vi "Stacking SSI.vi"(10 "Stacking SS State":T3, 11 "Robot Controls":T4) -> (3 "Stacking Actuators Out":T1)   [LabVIEW 2014]
uses:
  Robot Commands.ctl
  Stacking SS State.ctl
  Stacking SS Actuators.ctl
  <vilib>/Rock Robotics/WPI/Solenoid/WPI_SolenoidValue.ctl
  Global Variables/Settings.vi
  Global Variables/Lifter Sequences.vi
panel:
  out "Totes in Bot":i32
  # "Field Centric"
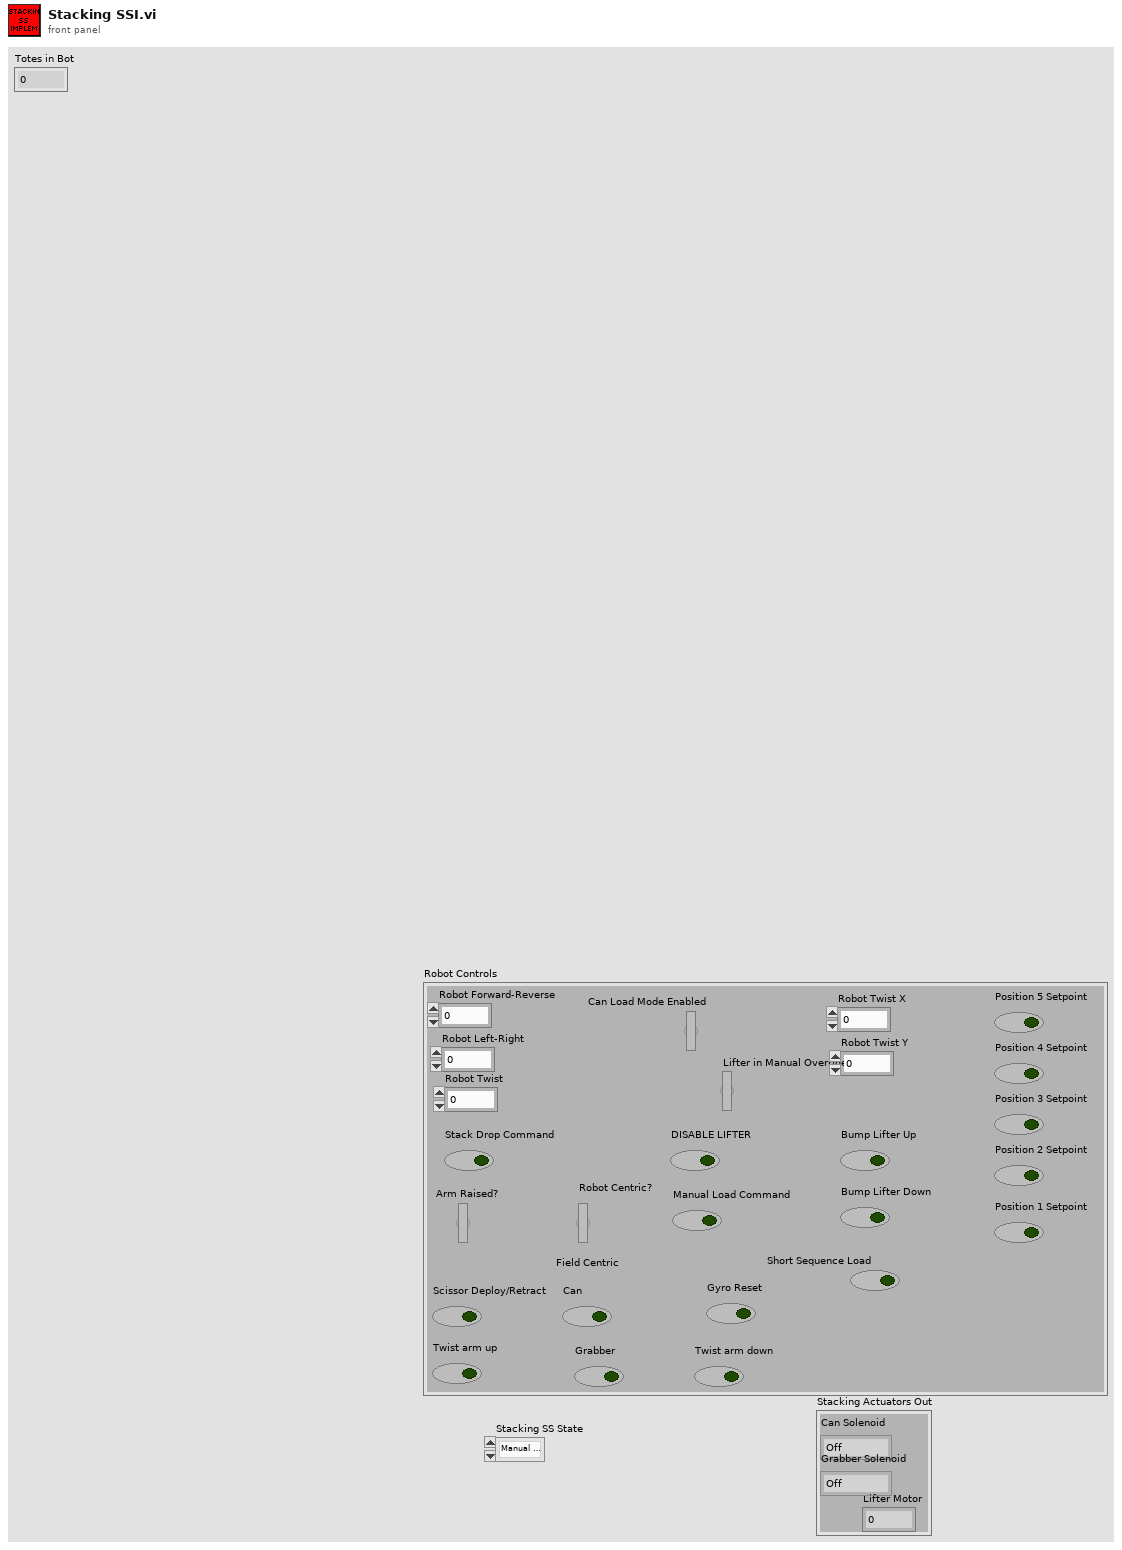
[diagram p1: front panel]
types:
  T1 = typedef "Stacking SS Actuators.ctl" = cluster{"Can Solenoid":T2, "Lifter Motor":dbl, "Grabber Solenoid":T2}
  T2 = typedef "WPI_SolenoidValue.ctl" = enum16{"Off", "On", "Forward", "Reverse"}
  T3 = typedef "Stacking SS State.ctl" = enum16{"Manual Load", "Manual Override"}
  T4 = typedef "Robot Commands.ctl" = cluster{"Robot Forward-Reverse":dbl, "Robot Left-Right":dbl, "Robot Twist":dbl, "Can Load Mode Enabled":bool, "Lifter in Manual Override?":bool, "Stack Drop Command":bool, "Arm Raised?":bool, "DISABLE LIFTER":bool, "Position 1 Setpoint":bool, "Position 2 Setpoint":bool, "Position 3 Setpoint":bool, "Position 4 Setpoint":bool, "Position 5 Setpoint":bool, "Bump Lifter Down":bool, "Bump Lifter Up":bool, "Manual Load Command":bool, "Robot Centric?":bool, "Scissor Deploy/Retract":bool, "Grabber":bool, "Can":bool, "Twist arm up":bool, "Gyro Reset":bool, "Twist arm down":bool, "Short Sequence Load":bool, "Robot Twist X":dbl, "Robot Twist Y":dbl}
  T5 = cluster{"Setpoint Commands":enum16{"No Op", "Setpoint 1", "Setpoint 2", "Setpoint 3", "Setpoint 4", "Setpoint 5"}[], "Setpoint Commands Wait for Input?":bool[], "Setpoint Commands Time Wait after setpoint reachd":i32[], "Can Solenoid Commands":enum16{"Disengaged", "Engaged"}[], "Grabber Solenoid Commands":enum16{"Disengaged", "Engaged"}[]}
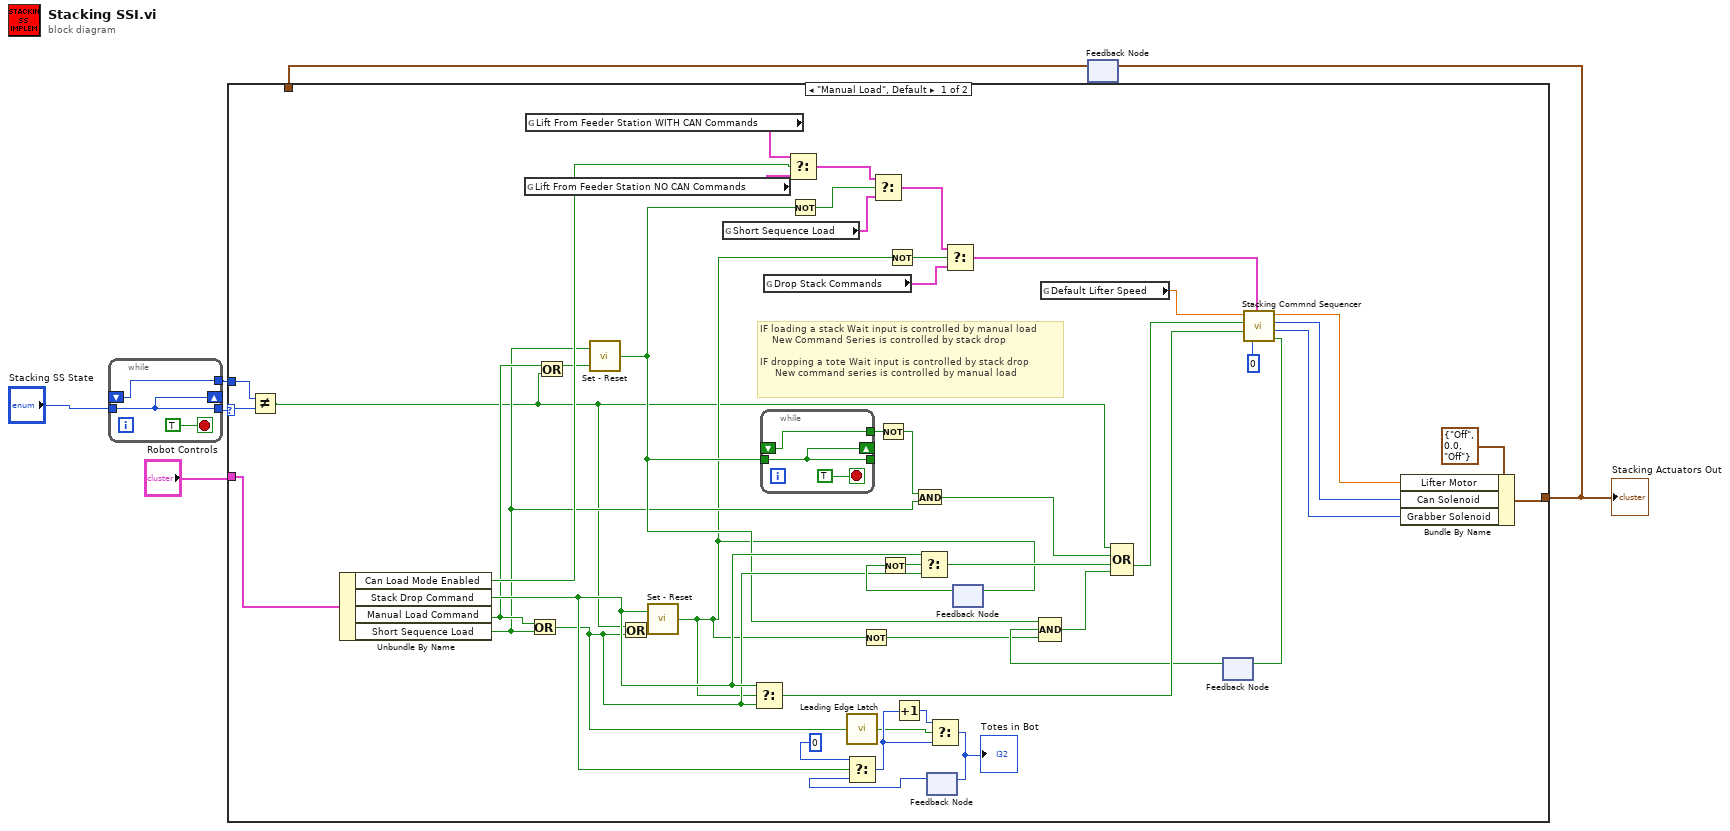
[diagram p0: block diagram]
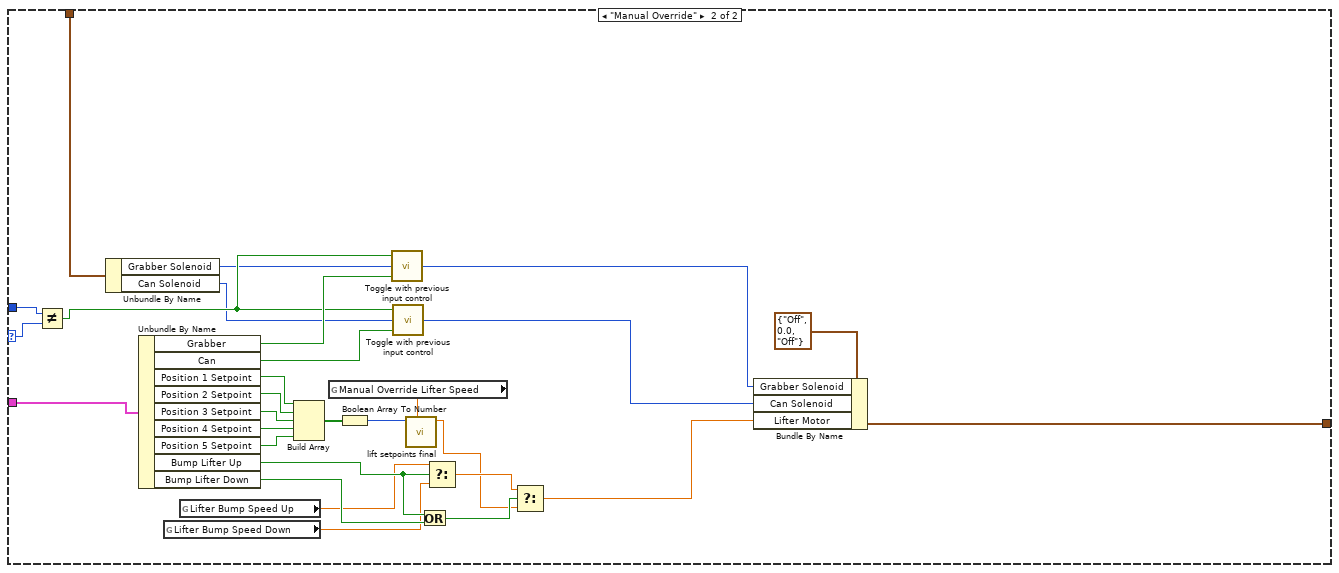
[diagram p2: hidden frame]
diagram:
  n1 = while {
    tunnel: "Stacking SS State" -> [w8]
    tunnel: [w8] -> w3
    shift-right: [w8] -> _
    shift-left: _ -> [w7]
    tunnel: [w7] -> w4
    stop <- TRUE stop-if-true
  }
  n2 = feedback #1() -> (w1:T1)  [unwired: 1 in]
  n3 = case shown="\"Manual Load\", Default" w3 {
    selector: w3 -> [w15 w67]
    tunnel: "Robot Controls" -> [w22 w88]
    tunnel: [w56 w74] -> w2
    tunnel: w4 -> [w14 w66]
    tunnel: w1 -> [_ w62]
    frame "Manual Load", Default {
      # "IF loading a stack Wait input is controlled by manual load\n    New Command Series is controlled by stack drop\n\nIF dropping a tote Wait input is controlled by stack drop\n     New command series is controlled by manual load"
      n4 = Not Equal?(x=w14, y=w15) -> (x != y?=w10:bool)
      n5 = Unbundle By Name(w22) -> ("Can Load Mode Enabled"=w53:bool, "Stack Drop Command"=w51:bool, "Manual Load Command"=w28:bool, "Short Sequence Load"=w25:bool)
      n6 = global read "Lifter Sequences.vi" "Lift From Feeder Station NO CAN Commands"() -> (w44:T5)
      n7 = global read "Lifter Sequences.vi" "Lift From Feeder Station WITH CAN Commands"() -> (w43:T5)
      n8 = Or(x=w28, y=w25) -> (x .or. y?=w36:bool)
      n9 = Or(x=w28, y=w10) -> (x .or. y?=w12:bool)
      n10 = call "Set - Reset.vi"("Reset"=w12, "Set"=w25) -> ("Output"=w26:bool)
      n11 = Or(x=w10, y=w36) -> (x .or. y?=w11:bool)
      n12 = call "Set - Reset.vi"("Reset"=w11, "Set"=w51) -> ("Output"=w18:bool)
      n13 = global read "Lifter Sequences.vi" "Short Sequence Load"() -> (w33:T5)
      n14 = Select(t=w51, s=w18, f=w36) -> (s? t:f=w32:bool)
      n15 = while {
        tunnel: w26 -> [w58]
        tunnel: [w58] -> _
        shift-right: [w58] -> _
        shift-left: _ -> [w57]
        tunnel: [w57] -> w24
        stop <- TRUE stop-if-true
      }
      n16 = global read "Lifter Sequences.vi" "Drop Stack Commands"() -> (w41:T5)
      n17 = Select(t=w43, s=w53, f=w44) -> (s? t:f=w34:T5)
      n18 = Not(x=w26) -> (.not. x?=w27:bool)
      n19 = call "Leading Edge Latch.vi"("Input"=w36) -> ("Output"=w39:bool)
      n20 = Not(x=w18) -> (.not. x?=w17:bool)
      n21 = Select(t=w34, s=w27, f=w33) -> (s? t:f=w35:T5)
      n22 = Not(x=w24) -> (.not. x?=w23:bool)
      n23 = Not(x=w18) -> (.not. x?=w40:bool)
      n24 = And(x=w23, y=w25) -> (x .and. y?=w16:bool)
      n25 = feedback #2() -> (w45:i32)  [unwired: 1 in]
      n26 = Select(t=0, s=w51, f=w45) -> (s? t:f=w47:i32)
      n27 = Increment(x=w47) -> (x+1=w48:i32)
      n28 = Select(t=w48, s=w39, f=w47) -> (s? t:f=w46:i32)
      "Totes in Bot" <- w46
      n29 = feedback-in #2(w46) -> ()
      n30 = Select(t=w35, s=w40, f=w41) -> (s? t:f=w50:T5)
      n31 = feedback #3() -> (w38:bool)  [unwired: 1 in]
      n32 = Not(x=w38) -> (.not. x?=w37:bool)
      n33 = Select(t=w51, s=w37, f=w36) -> (s? t:f=w42:bool)
      n34 = feedback-in #3(w18) -> ()
      n35 = global read "Settings.vi" "Default Lifter Speed"() -> (w13:dbl)
      n36 = feedback #4() -> (w30:bool)  [unwired: 1 in]
      n37 = Compound Arithmetic op=AND(w26, w30, w17) -> (w29:bool)
      n38 = Compound Arithmetic op=OR(w10, w16, w42, w29) -> (w52:bool)
      n39 = call "Stacking Commnd Sequencer.vi"("Lifter Commands"=w50, "Command Series Start Index"=0, "Wait Input"=w32, "New Command Series"=w52, "Set Motor Speed"=w13) -> ("Series Finished"=w31:bool, "Grabber Solenoid"=w21:T2, "Can Solenoid"=w20:T2, "Motor Speed"=w19:dbl)
      n40 = feedback-in #4(w31) -> ()
      n41 = Bundle By Name(cluster=T1 {"Can Solenoid"=enum."Off", "Lifter Motor"=0.0, "Grabber Solenoid"=enum."Off"} ("Stacking Actuators Out"), "Lifter Motor"=w19, "Can Solenoid"=w20, "Grabber Solenoid"=w21) -> (w56:T1)
    }
    frame "Manual Override" {
      n42 = Not Equal?(x=w66, y=w67) -> (x != y?=w65:bool)
      n43 = Unbundle By Name(w62) -> ("Grabber Solenoid"=w60:T2, "Can Solenoid"=w61:T2)
      n44 = Unbundle By Name(w88) -> ("Grabber"=w69:bool, "Can"=w68:bool, "Position 1 Setpoint"=w87:bool, "Position 2 Setpoint"=w86:bool, "Position 3 Setpoint"=w85:bool, "Position 4 Setpoint"=w84:bool, "Position 5 Setpoint"=w83:bool, "Bump Lifter Up"=w81:bool, "Bump Lifter Down"=w80:bool)
      n45 = global read "Settings.vi" "Lifter Bump Speed Down"() -> (w71:dbl)
      n46 = global read "Settings.vi" "Lifter Bump Speed Up"() -> (w72:dbl)
      n47 = Build Array(w87, w86, w85, w84, w83) -> (w82:bool[])
      n48 = global read "Settings.vi" "Manual Override Lifter Speed"() -> (w73:dbl)
      n49 = Boolean Array To Number(Boolean array=w82) -> (number=w70:u32)
      n50 = call "Toggle with previous input control.vi"("Control"=w69, "Previous Input"=w60, "Reset to Previous Input?"=w65) -> ("Output"=w64:T2)
      n51 = call "Toggle with previous input control.vi"("Control"=w68, "Previous Input"=w61, "Reset to Previous Input?"=w65) -> ("Output"=w63:T2)
      n52 = call "lift setpoints final.vi"("Set Motor Speed"=w73, "Requested Position\n(0, 1, 2, 4, 8, 16)"=w70) -> ("Motor Speed"=w77:dbl)  [unwired: 8 in, 1 out]
      n53 = Or(x=w81, y=w80) -> (x .or. y?=w79:bool)
      n54 = Select(t=w72, s=w81, f=w71) -> (s? t:f=w78:dbl)
      n55 = Select(t=w78, s=w79, f=w77) -> (s? t:f=w76:dbl)
      n56 = Bundle By Name(cluster=T1 {"Can Solenoid"=enum."Off", "Lifter Motor"=0.0, "Grabber Solenoid"=enum."Off"} ("Cluster"), "Grabber Solenoid"=w64, "Can Solenoid"=w63, "Lifter Motor"=w76) -> (w74:T1)
    }
  }
  "Stacking Actuators Out" <- w2
  n57 = feedback-in #1(w2) -> ()
